vi "2.1.vi"() -> ()   [LabVIEW 2017]
panel:
  out "y":dbl
  in  "b":dbl
  in  "x":dbl
  in  "k\nk":dbl
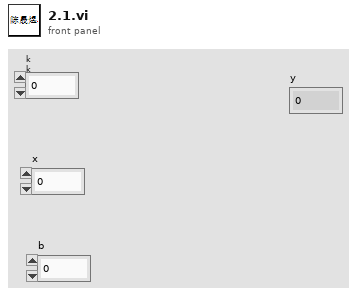
[diagram p1: front panel]
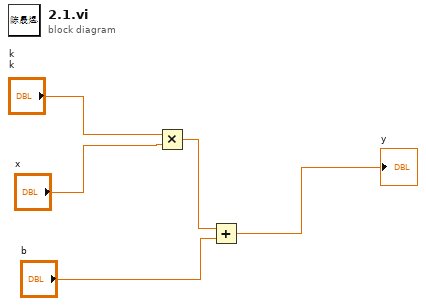
[diagram p0: block diagram]
diagram:
  n1 = Multiply(x="k\nk", y="x") -> (x*y=w3:dbl)
  n2 = Add(x=w3, y="b") -> (x+y=→"y":dbl)
